vi "Get Cooler Status.vi"(8 "error in (no error)":errorcluster, 11 "Cooler in":refnum<class "Simulated_Cooler.lvclass">) -> (0 "error out":errorcluster, 3 "Cooler out":refnum<class "Simulated_Cooler.lvclass">)   [LabVIEW 2018, in "Simulated_Cooler.lvclass"]
uses:
  Simulated_Cooler.lvclass
  <userlib>/atmcd32d.llb/Error Code Enum typedef.ctl
  Simulated_Cooler.lvclass/Simulated_Cooler.ctl
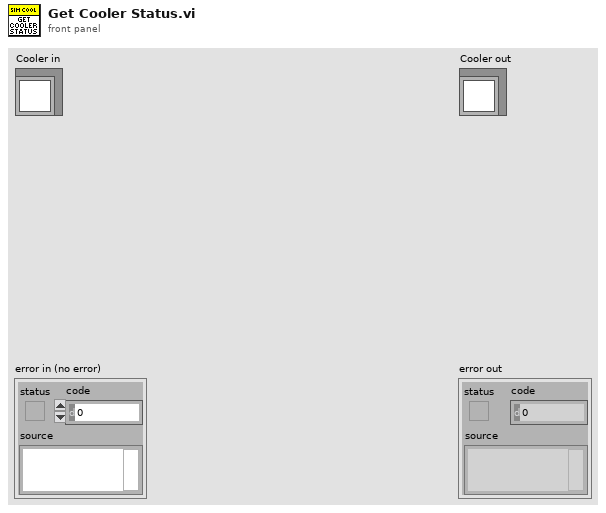
[diagram p1: front panel]
types:
  T1 = typedef "Error Code Enum typedef.ctl" = enum32{"N/A (0)", "DRV_ERROR_CODES", "DRV_SUCCESS", "DRV_VXDNOTINSTALLED", "DRV_ERROR_SCAN", "DRV_ERROR_CHECK_SUM", "DRV_ERROR_FILELOAD", "DRV_UNKNOWN_FUNC", "DRV_ERROR_VXD_INIT", "DRV_ERROR_ADDRESS", "DRV_ERROR_PAGELOCK", "DRV_ERROR_PAGEUNLOCK", "DRV_ERROR_BOARDTEST", "DRV_ERROR_ACK", "DRV_ERROR_UP_FIFO", "DRV_ERROR_PATTERN", "N/A (16)", "DRV_ACQUISITION_ERRORS", "DRV_ACQ_BUFFER", "DRV_ACQ_DOWNFIFO_FULL", "DRV_PROC_UNKONWN_INSTRUCTION", "DRV_ILLEGAL_OP_CODE", "DRV_KINETIC_TIME_NOT_MET", "DRV_ACCUM_TIME_NOT_MET", "DRV_NO_NEW_DATA", "N/A (25)", "DRV_SPOOLERROR", "N/A (27)", "N/A (28)", "N/A (29)", "N/A (30)", "N/A (31)", "N/A (32)", "DRV_TEMPERATURE_CODES", "DRV_TEMPERATURE_OFF", "DRV_TEMPERATURE_NOT_STABILIZED", "DRV_TEMPERATURE_STABILIZED", "DRV_TEMPERATURE_NOT_REACHED", "DRV_TEMPERATURE_OUT_RANGE", "DRV_TEMPERATURE_NOT_SUPPORTED", "DRV_TEMPERATURE_DRIFT", "N/A (41)", "N/A (42)", "N/A (43)", "N/A (44)", "N/A (45)", "N/A (46)", "N/A (47)", "N/A (48)", "DRV_GENERAL_ERRORS", "DRV_INVALID_AUX", "DRV_COF_NOTLOADED", "DRV_FPGAPROG", "DRV_FLEXERROR", "DRV_GPIBERROR", "N/A (55)", "N/A (56)", "N/A (57)", "N/A (58)", "N/A (59)", "N/A (60)", "N/A (61)", "N/A (62)", "N/A (63)", "DRV_DATATYPE", "DRV_DRIVER_ERRORS", "DRV_P1INVALID", "DRV_P2INVALID", "DRV_P3INVALID", "DRV_P4INVALID", "DRV_INIERROR", "DRV_COFERROR", "DRV_ACQUIRING", "DRV_IDLE", "DRV_TEMPCYCLE", "DRV_NOT_INITIALIZED", "DRV_P5INVALID", "DRV_P6INVALID", "DRV_INVALID_MODE", "DRV_INVALID_FILTER", "DRV_I2CERRORS", "DRV_I2CDEVNOTFOUND", "DRV_I2CTIMEOUT", "DRV_P7INVALID", "N/A (84)", "N/A (85)", "N/A (86)", "N/A (87)", "N/A (88)", "N/A (89)", "DRV_IOCERROR", "DRV_VRMVERSIONERROR"}
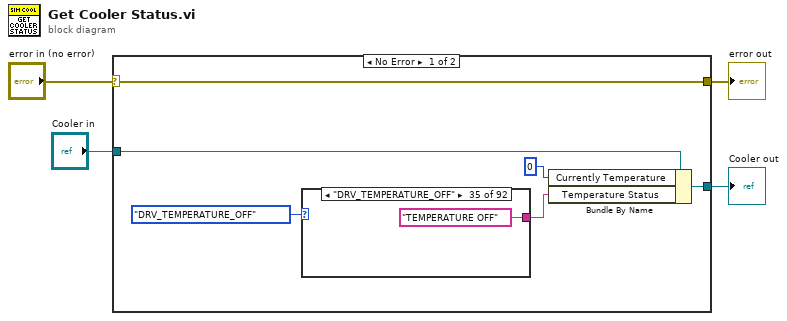
[diagram p0: block diagram]
diagram:
  n1 = case shown="No Error" "error in (no error)" {
    selector: "error in (no error)" -> [w10 w16]
    tunnel: [w10 w16] -> w3
    tunnel: [w7 w15] -> w1
    tunnel: "Cooler in" -> [w9 w15]
    frame No Error {
      n2 = case shown="\"DRV_TEMPERATURE_OFF\"" Error_Code_Enum_typedef."DRV_TEMPERATURE_OFF" ("status") {
        tunnel: [_ _ _ _ _ _ _ _ _ _ _ _ _ _ _ _ _ _ _ _ _ _ _ _ _ _ _ _ _ _ _ _ _ _ "TEMPERATURE OFF" "TEMPERATURE NOT STABILIZED" "TEMPERATURE STABILIZED" "TEMPERATURE NOT REACHED" _ _ _ _ _ _ _ _ _ _ _ _ _ _ _ _ _ _ _ _ _ _ _ _ _ _ _ _ _ _ _ _ _ _ _ _ _ _ _ _ _ _ _ _ _ _ _ _ _ _ _ _ _ _] -> w8
        frame "N/A (0)", Default {
        }
        frame "DRV_ERROR_CODES" {
        }
        frame "DRV_SUCCESS" {
        }
        frame "DRV_VXDNOTINSTALLED" {
        }
        frame "DRV_ERROR_SCAN" {
        }
        frame "DRV_ERROR_CHECK_SUM" {
        }
        frame "DRV_ERROR_FILELOAD" {
        }
        frame "DRV_UNKNOWN_FUNC" {
        }
        frame "DRV_ERROR_VXD_INIT" {
        }
        frame "DRV_ERROR_ADDRESS" {
        }
        frame "DRV_ERROR_PAGELOCK" {
        }
        frame "DRV_ERROR_PAGEUNLOCK" {
        }
        frame "DRV_ERROR_BOARDTEST" {
        }
        frame "DRV_ERROR_ACK" {
        }
        frame "DRV_ERROR_UP_FIFO" {
        }
        frame "DRV_ERROR_PATTERN" {
        }
        frame "N/A (16)" {
        }
        frame "DRV_ACQUISITION_ERRORS" {
        }
        frame "DRV_ACQ_BUFFER" {
        }
        frame "DRV_ACQ_DOWNFIFO_FULL" {
        }
        frame "DRV_PROC_UNKONWN_INSTRUCTION" {
        }
        frame "DRV_ILLEGAL_OP_CODE" {
        }
        frame "DRV_KINETIC_TIME_NOT_MET" {
        }
        frame "DRV_ACCUM_TIME_NOT_MET" {
        }
        frame "DRV_NO_NEW_DATA" {
        }
        frame "N/A (25)" {
        }
        frame "DRV_SPOOLERROR" {
        }
        frame "N/A (27)" {
        }
        frame "N/A (28)" {
        }
        frame "N/A (29)" {
        }
        frame "N/A (30)" {
        }
        frame "N/A (31)" {
        }
        frame "N/A (32)" {
        }
        frame "DRV_TEMPERATURE_CODES" {
        }
        frame "DRV_TEMPERATURE_OFF" {
        }
        frame "DRV_TEMPERATURE_NOT_STABILIZED" {
        }
        frame "DRV_TEMPERATURE_STABILIZED" {
        }
        frame "DRV_TEMPERATURE_NOT_REACHED" {
        }
        frame "DRV_TEMPERATURE_OUT_RANGE" {
        }
        frame "DRV_TEMPERATURE_NOT_SUPPORTED" {
        }
        frame "DRV_TEMPERATURE_DRIFT" {
        }
        frame "N/A (41)" {
        }
        frame "N/A (42)" {
        }
        frame "N/A (43)" {
        }
        frame "N/A (44)" {
        }
        frame "N/A (45)" {
        }
        frame "N/A (46)" {
        }
        frame "N/A (47)" {
        }
        frame "N/A (48)" {
        }
        frame "DRV_GENERAL_ERRORS" {
        }
        frame "DRV_INVALID_AUX" {
        }
        frame "DRV_COF_NOTLOADED" {
        }
        frame "DRV_FPGAPROG" {
        }
        frame "DRV_FLEXERROR" {
        }
        frame "DRV_GPIBERROR" {
        }
        frame "N/A (55)" {
        }
        frame "N/A (56)" {
        }
        frame "N/A (57)" {
        }
        frame "N/A (58)" {
        }
        frame "N/A (59)" {
        }
        frame "N/A (60)" {
        }
        frame "N/A (61)" {
        }
        frame "N/A (62)" {
        }
        frame "N/A (63)" {
        }
        frame "DRV_DATATYPE" {
        }
        frame "DRV_DRIVER_ERRORS" {
        }
        frame "DRV_P1INVALID" {
        }
        frame "DRV_P2INVALID" {
        }
        frame "DRV_P3INVALID" {
        }
        frame "DRV_P4INVALID" {
        }
        frame "DRV_INIERROR" {
        }
        frame "DRV_COFERROR" {
        }
        frame "DRV_ACQUIRING" {
        }
        frame "DRV_IDLE" {
        }
        frame "DRV_TEMPCYCLE" {
        }
        frame "DRV_NOT_INITIALIZED" {
        }
        frame "DRV_P5INVALID" {
        }
        frame "DRV_P6INVALID" {
        }
        frame "DRV_INVALID_MODE" {
        }
        frame "DRV_INVALID_FILTER" {
        }
        frame "DRV_I2CERRORS" {
        }
        frame "DRV_I2CDEVNOTFOUND" {
        }
        frame "DRV_I2CTIMEOUT" {
        }
        frame "DRV_P7INVALID" {
        }
        frame "N/A (84)" {
        }
        frame "N/A (85)" {
        }
        frame "N/A (86)" {
        }
        frame "N/A (87)" {
        }
        frame "N/A (88)" {
        }
        frame "N/A (89)" {
        }
        frame "DRV_IOCERROR" {
        }
        frame "DRV_VRMVERSIONERROR" {
        }
      }
      n3 = Bundle By Name(cluster=w9, "Currently Temperature"=i16 0, "Temperature Status"=w8) -> (w7:refnum<class "Simulated_Cooler.lvclass">)
    }
    frame Error {
    }
  }
  "error out" <- w3
  "Cooler out" <- w1
